vi "oa_Check Samples-Rev Setting for Buffer VI.vi"(8 "error in (no error)":errorcluster, 10 "buffer settings":T2, 11 "position info":T1) -> (0 "error out":errorcluster)   [LabVIEW 2017, in "SoundVib_OAUtility.lvlib"]
uses:
  <vilib>/addons/Sound and Vibration/Order Analysis/Utility/SoundVib_OAUtility.lvlib
  <vilib>/addons/Sound and Vibration/Order Analysis/Utility/SubVIs/oa_Buffer Settings.ctl
  <vilib>/addons/Sound and Vibration/Order Analysis/Misc/OAT Position Info.ctl
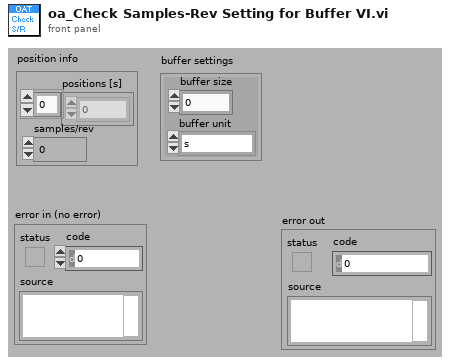
[diagram p1: front panel]
types:
  T1 = typedef "OAT Position Info.ctl" = cluster{"positions [s]":dbl[], "samples/rev":dbl}
  T2 = typedef "SoundVib_OAUtility.lvlib/oa_Buffer Settings.ctl" = cluster{"buffer size":dbl, "buffer unit":enum16{"s", "revolution", "# of samples"}}
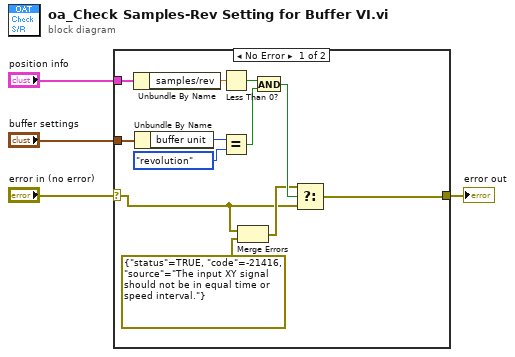
[diagram p0: block diagram]
diagram:
  n1 = case shown="No Error" "error in (no error)" {
    selector: "error in (no error)" -> [w6 w17]
    tunnel: "position info" -> [w16 _]
    tunnel: "buffer settings" -> [w15 _]
    tunnel: [w8 w17] -> w1
    frame No Error {
      n2 = Unbundle By Name(w16) -> ("samples/rev"=w14:dbl)
      n3 = Unbundle By Name(w15) -> ("buffer unit"=w13:enum16{"s", "revolution", "# of samples"})
      n4 = Less Than 0?(x=w14) -> (x < 0?=w11:bool)
      n5 = Equal?(x=w13, y=enum16{"s", "revolution", "# of samples"}."revolution" ("buffer unit")) -> (x = y?=w10:bool)
      n6 = Merge Errors(w6, errorcluster {"status"=TRUE, "code"=-21416, "source"="The input XY signal should not be in equal time or speed interval."} ("f")) -> (w7:errorcluster)
      n7 = And(x=w11, y=w10) -> (x .and. y?=w9:bool)
      n8 = Select(t=w7, s=w9, f=w6) -> (s? t:f=w8:errorcluster)
    }
    frame Error {
    }
  }
  "error out" <- w1
